vi "Matrix MinMax By Row Or Column.vi"(8 "By column?":bool, 11 "2D Array":dbl[][](array[numeric])) -> (0 "Min Indices":i32[](array[numeric]), 1 "Min Vector":dbl[](array[numeric]), 2 "Max Indices":i32[](array[numeric]), 3 "Max Vector":dbl[](array[numeric]))   [LabVIEW 2020]
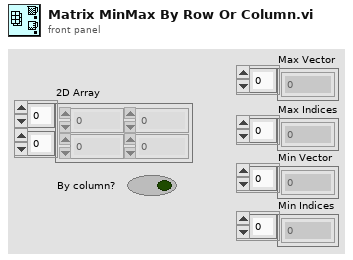
[diagram p1: front panel]
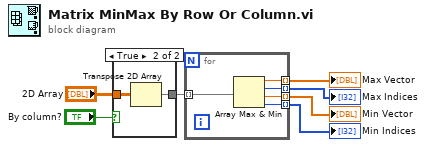
[diagram p0: block diagram]
diagram:
  n1 = case shown="True" "By column?" {
    tunnel: "2D Array" -> [w8 w10]
    tunnel: [w8 w9] -> w5
    frame False {
    }
    frame True {
      n2 = Transpose 2D Array(2D array=w10) -> (transposed array=w9:dbl[][])
    }
  }
  n3 = for {
    tunnel: w5 -> [w15] mode=indexing
    tunnel: [w14] -> w6 mode=indexing
    tunnel: [w13] -> w4 mode=indexing
    tunnel: [w12] -> w3 mode=indexing
    tunnel: [w11] -> w2 mode=indexing
    n4 = Array Max & Min(array=w15) -> (max value=w14:dbl, max index (indices)=w13:i32, min value=w12:dbl, min index (indices)=w11:i32)
  }
  "Max Vector" <- w6
  "Max Indices" <- w4
  "Min Vector" <- w3
  "Min Indices" <- w2
